vi "Pre Launch Init.vi"(11 "PLC Sim Controller Actor in":refnum<class "PLC Sim Controller Actor.lvclass">) -> (0 "error out":errorcluster, 3 "PLC Sim Controller Actor out":refnum<class "PLC Sim Controller Actor.lvclass">)   [LabVIEW 2019, in "PLC Sim Controller Actor.lvlib" / "PLC Sim Controller Actor.lvclass"]
doc: "(<B>Filename</B>: Actor Framework.lvlib:Actor.lvclass:Pre Launch Init.vi)\n\nDefines behavior that occurs after the Launch Nested Actor method is invoked but before the actor's Actor Core method begins running.\n\nBy default, this method does nothing. A descendant class may override it to define behavior."
uses:
  PLC Sim Controller Actor.lvclass
  PLC Sim Controller Actor.lvclass/PLC Sim Controller Actor.ctl
  <vilib>/ActorFramework/Actor/Actor.lvclass
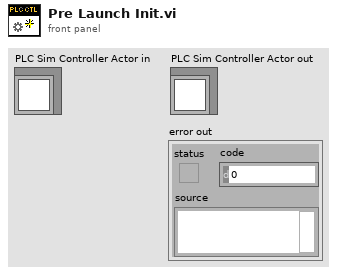
[diagram p1: front panel]
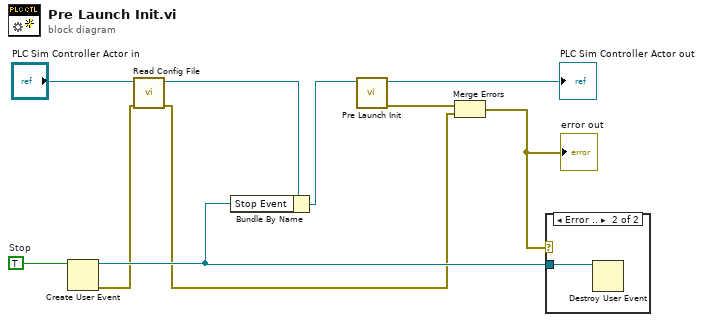
[diagram p0: block diagram]
diagram:
  w9 = TRUE  # Stop
  n1 = Create User Event(user event datatype=w9) -> (user event=w5:refnum<user-event>, error out=w2:errorcluster)  [unwired: 1 in]
  n2 = call "Read Config File.vi"("error in (no error)"=w2, "SM EOL Station Actor in"="PLC Sim Controller Actor in") -> ("error out"=w1:errorcluster, "SM EOL Station Actor out"=w3:refnum<class "PLC Sim Controller Actor.lvclass">)  [unwired: 8 in]
  n3 = Bundle By Name(cluster=w3, "Stop Event"=w5) -> (w8:refnum<class "PLC Sim Controller Actor.lvclass">)
  n4 = call-parent "Pre Launch Init.vi"("Actor in"=w8) -> ("error out"=w7:errorcluster, "Actor out"=→"PLC Sim Controller Actor out":refnum<class "PLC Sim Controller Actor.lvclass">)  [unwired: 9 in]
  n5 = Merge Errors(w7, w1) -> (w6:errorcluster)
  "error out" <- w6
  n6 = case shown="Error .." w6 {
    tunnel: w5 -> [_ w11]
    frame No Error {
    }
    frame Error {
      n7 = Destroy User Event(user event=w11) -> ()  [unwired: 1 in, 1 out]
    }
  }
